vi "Enum to Data Type.vi"(10 "Variable Data Type":T1) -> (2 "Variant":variant)   [LabVIEW 2015]
doc: "Convert SV data type enum to an enum accepted by the shared variable API."
uses:
  Type Defs/Variable Data Type.ctl
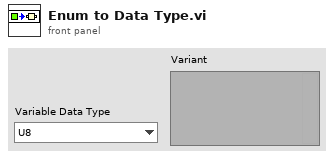
[diagram p1: front panel]
types:
  T1 = typedef "Variable Data Type.ctl" = enum16{"U8", "U16", "U32", "U64", "I8", "I16", "I32", "I64", "Single", "Double", "Boolean", "String"}
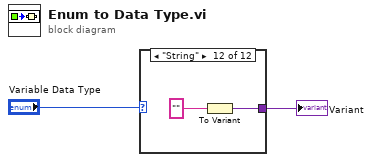
[diagram p0: block diagram]
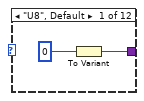
[diagram p2: hidden frame]
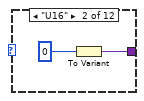
[diagram p3: hidden frame]
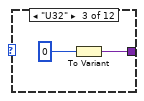
[diagram p4: hidden frame]
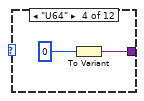
[diagram p5: hidden frame]
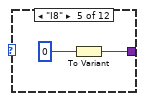
[diagram p6: hidden frame]
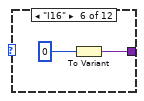
[diagram p7: hidden frame]
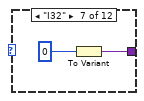
[diagram p8: hidden frame]
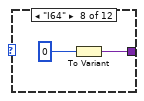
[diagram p9: hidden frame]
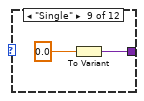
[diagram p10: hidden frame]
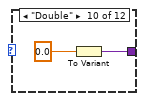
[diagram p11: hidden frame]
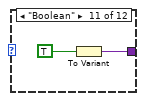
[diagram p12: hidden frame]
diagram:
  n1 = case shown="\"String\"" "Variable Data Type" {
    tunnel: [w3 w5 w7 w9 w11 w13 w15 w17 w19 w21 w23 w25] -> w1
    frame "U8", Default {
      n2 = To Variant(anything=u8 0) -> (Variant=w3:variant)
    }
    frame "U16" {
      n3 = To Variant(anything=u16 0) -> (Variant=w5:variant)
    }
    frame "U32" {
      n4 = To Variant(anything=u32 0) -> (Variant=w7:variant)
    }
    frame "U64" {
      n5 = To Variant(anything=u64 0) -> (Variant=w9:variant)
    }
    frame "I8" {
      n6 = To Variant(anything=i8 0) -> (Variant=w11:variant)
    }
    frame "I16" {
      n7 = To Variant(anything=i16 0) -> (Variant=w13:variant)
    }
    frame "I32" {
      n8 = To Variant(anything=0) -> (Variant=w15:variant)
    }
    frame "I64" {
      n9 = To Variant(anything=i64 0) -> (Variant=w17:variant)
    }
    frame "Single" {
      n10 = To Variant(anything=sgl 0.0) -> (Variant=w19:variant)
    }
    frame "Double" {
      n11 = To Variant(anything=0.0) -> (Variant=w21:variant)
    }
    frame "Boolean" {
      n12 = To Variant(anything=TRUE) -> (Variant=w23:variant)
    }
    frame "String" {
      n13 = To Variant(anything="") -> (Variant=w25:variant)
    }
  }
  "Variant" <- w1
